vi "TDC_Prototype.vi"() -> ()   [LabVIEW 2025]
uses:
  Labview-File/STM-Auto-Project Testing/STM-Auto-Project (Trial 2)/QMH CTLS/Scan_Params (QMH).ctl
  TDC_SubVI/TEMP_SWEEPER.ctl
  TDC_SubVI/Temp Cntrl.ctl
  Downloads/OneDrive_2025-11-26 (2)/Magnetic Drift Correction/XY_Coords(Final).ctl
panel:
  out "Z-Controller on/off status 2":bool
  out "Translation (m) 2":T1
  out "Final coordinates (m)  2":cluster{"Xc":sgl, "Yc":sgl} {"Yc" format="%.4p"; "Xc" format="%.4p"}
  out "Initial coordinates (m)  2":cluster{"Xc":sgl, "Yc":sgl} {"Yc" format="%.4p"; "Xc" format="%.4p"}
  out "Current Temp":dbl format="%#.5f"
  out "Temp. Array":dbl[](array[numeric])
  out "Z-Controller on/off status":bool
  in  "Field and Temp Range":T2={"VISA (Magnet)"="COM4", "Fields(T)"=[], "Temps(K)"=[], "VISA (Temp) "="Lakeshore_Model_350"}
  out "error out":errorcluster
  in  "Serial Configuration":T3={"Baud Rate"=57600, "Parity"=1, "Data Bits"=7, "Stop Bits"=10, "Flow Control"=0}
  out "Current Index":i32
  out "Translation (m)":T1
  out "Final coordinates (m)":cluster{"Xc":sgl, "Yc":sgl} {"Yc" format="%.4p"; "Xc" format="%.4p"}
  out "Initial coordinates (m)":cluster{"Xc":sgl, "Yc":sgl} {"Yc" format="%.4p"; "Xc" format="%.4p"}
  in  "stop":bool
  in  "Start":bool
  # "Main goals,\n\nSet base line: Do initial bias and scan\n\nChange temp: Init temp, temp on, temp stab,\n\nInter scan, move frame, final scan, bias shit,\n\nNext temp? Prep next field though reinialization, determine if higher range is needed, apply field by changing setpoint\n\nInter scan, move frame, final scan, bias shit,"
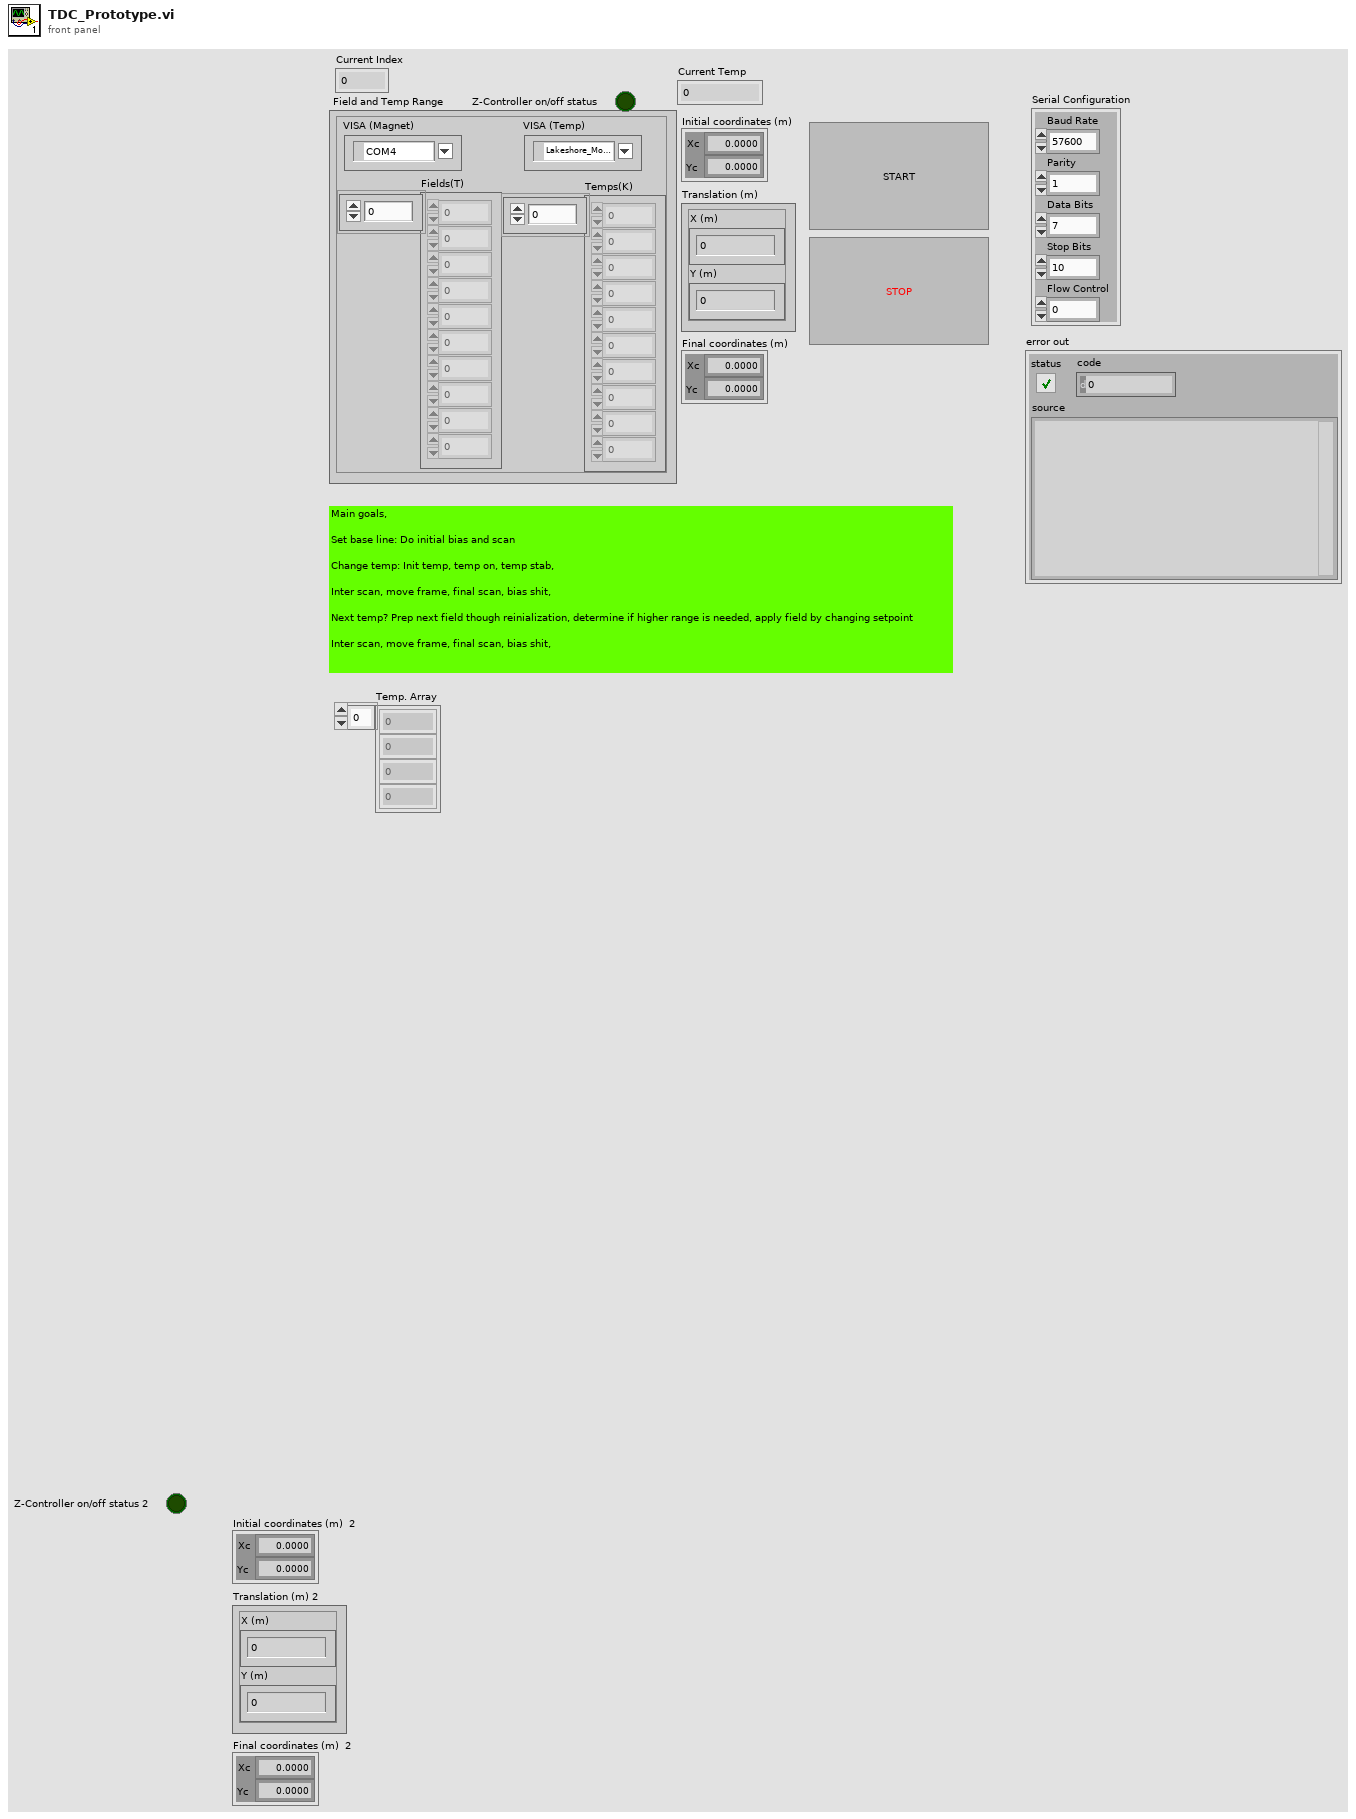
[diagram p1: front panel]
types:
  T1 = typedef "XY_Coords(Final).ctl" = cluster{"X (m)":dbl, "Y (m)":dbl}
  T2 = cluster{"VISA (Magnet)":refnum<visa-resource-name>, "Fields(T)":dbl[], "Temps(K)":dbl[], "VISA (Temp) ":refnum<visa-resource-name>}
  T3 = cluster{"Baud Rate":u32, "Parity":u16, "Data Bits":u16, "Stop Bits":u16, "Flow Control":u16}
  T4 = enum16{"1. BIAS", "2. INIT_SCAN", "3. SCAN_IDLE", "4. INTER_SCAN", "5. NEW_COORDS_&_FRAME", "6. FINAL_SCAN", "7. POLL_BIAS", "8. Z-CONT.", "9. STOP"}
  T5 = enum16{"SET TEMP", "SWEEP IDLE", "NEXT TEMP", "SWEEP DONE"}
  T6 = enum16{"1. INIT TEMP", "2. TC ON", "3. POLL_TEMPS", "4. TEMP_STAB", "5. TC IDLE", "6. APPLY NEXT TEMP", "7. TC OFF (Reset)"}
  T7 = typedef "Temp Cntrl.ctl" = cluster{"Range (0:Off)":u16, "Manual Output (0.00 %)":dbl, "Rate (D) (0.0 %)":dbl, "Reset (I) (20.0)":dbl, "Gain (P) (50.0)":dbl, "Power Up Enable (F: Disable)":bool, "Max User Current (2.000)":dbl, "Heater Resistance (1:25 Ohms)":u16, "Max Current (0:User Specified)":u16, "Heater Out Display (1:Current)":u16, "Mode (0:Off)":u16, "Input (0:None)":u16, "Target Temp (K)":dbl, "Serial Configuration":cluster{"Baud Rate":u32, "Parity":u16, "Data Bits":u16, "Stop Bits":u16, "Flow Control":u16}, "VISA resource name":refnum<visa-resource-name>, "Configure Control Parameters (0: Configure)":u16, "Enable Setpoint (F:Disable)":bool, "Input (0:A)":u16, "Data Source (0:Kelvin)":u16, "Output's Control Loop (1:1)":u16, "STND DEV Threshold ":dbl, "Mean Tolerance ":dbl, "Current State":enum16{"1. INIT TEMP", "2. TC ON", "3. POLL_TEMPS", "4. TEMP_STAB", "5. TC IDLE", "6. APPLY NEXT TEMP", "7. TC OFF (Reset)"}}
  T8 = typedef "TEMP_SWEEPER.ctl" = cluster{"Temps(K)":dbl[], "Sweep States":enum16{"SET TEMP", "SWEEP IDLE", "NEXT TEMP", "SWEEP DONE"}}
  T9 = typedef "Scan_Params (QMH).ctl" = cluster{"Setpoint (I)":dbl[], "Bias (V)":dbl[], "Number of scans":u8, "Port number (3364)":u32, "Avoid zero threshold (V)":dbl, "Current State":enum16{"1. BIAS", "2. INIT_SCAN", "3. SCAN_IDLE", "4. INTER_SCAN", "5. NEW_COORDS_&_FRAME", "6. FINAL_SCAN", "7. STOP"}}
  T10 = enum16{"1. BIAS", "2. INIT_SCAN", "3. SCAN_IDLE", "4. INTER_SCAN", "5. NEW_COORDS_&_FRAME", "6. FINAL_SCAN", "7. STOP"}
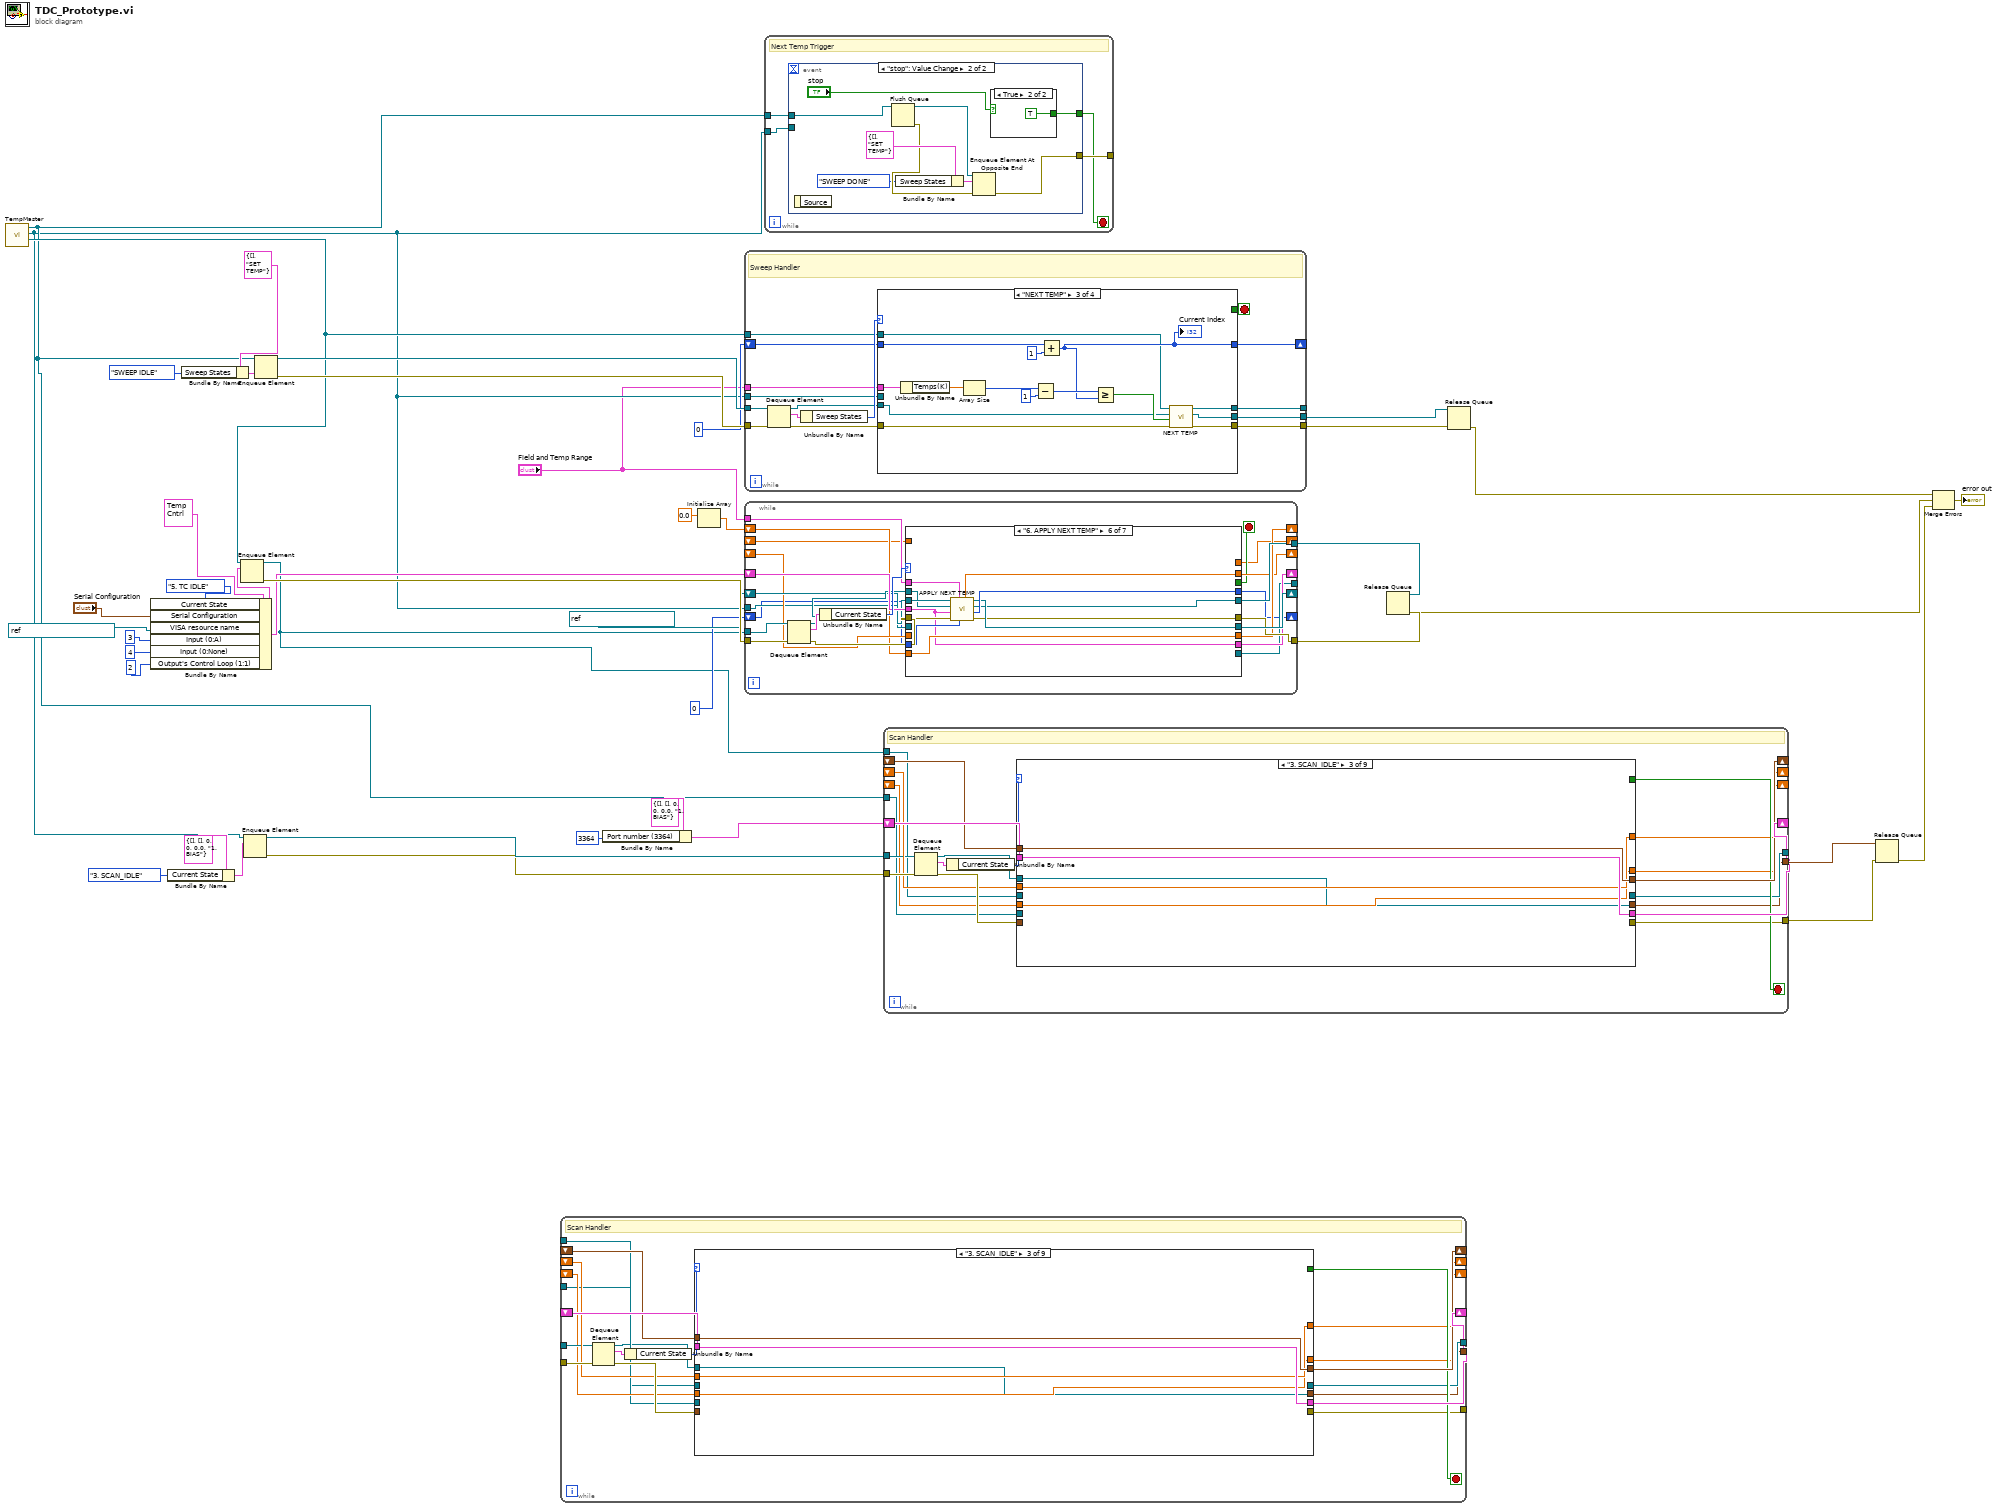
[diagram p0: block diagram]
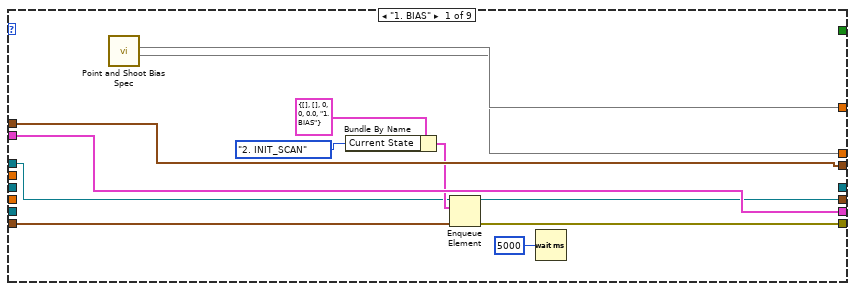
[diagram p2: hidden frame]
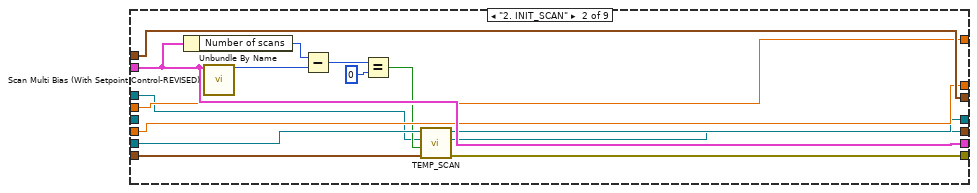
[diagram p3: hidden frame]
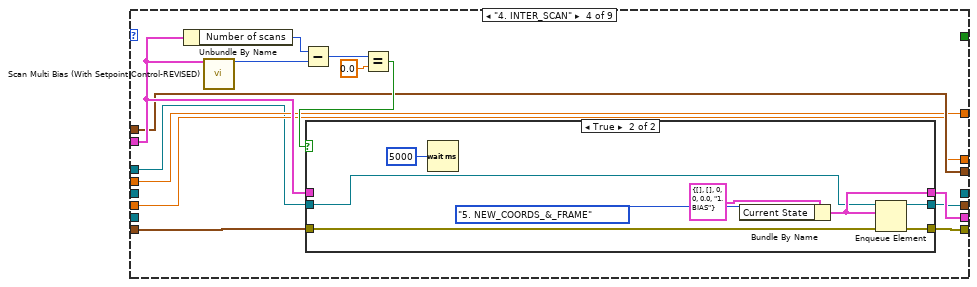
[diagram p4: hidden frame]
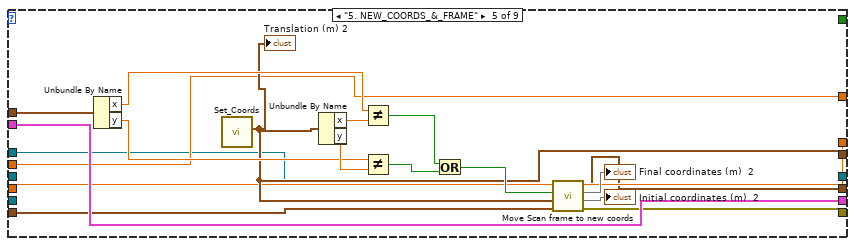
[diagram p6: hidden frame]
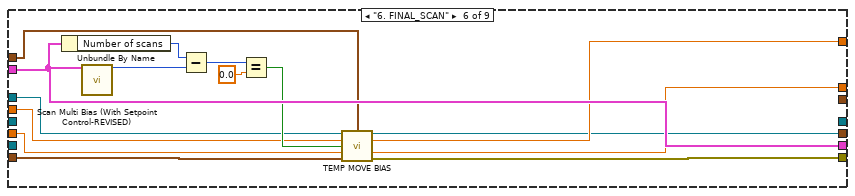
[diagram p7: hidden frame]
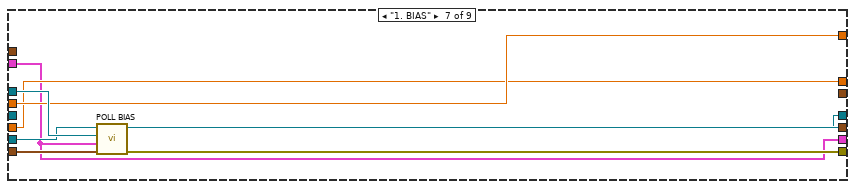
[diagram p8: hidden frame]
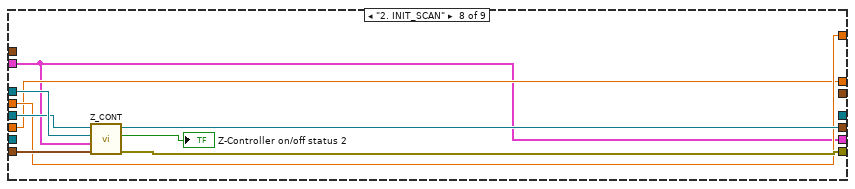
[diagram p9: hidden frame]
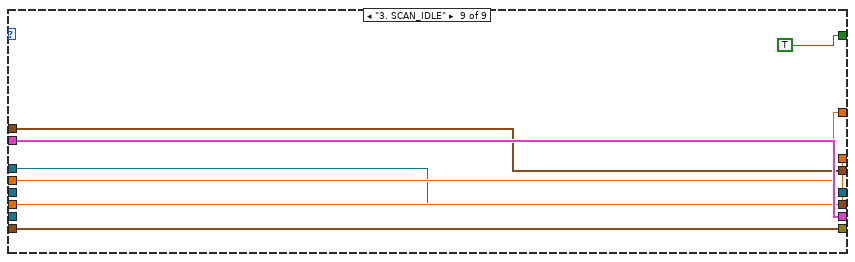
[diagram p10: hidden frame]
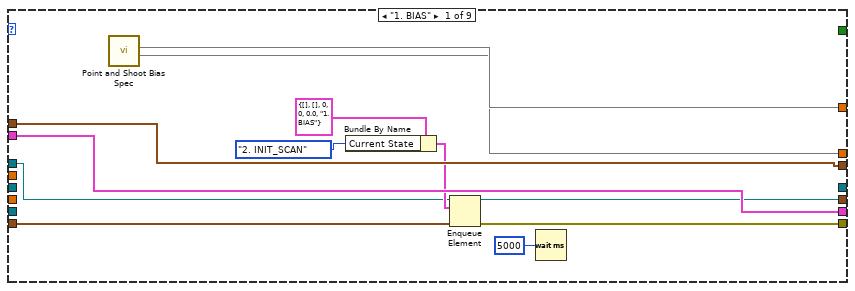
[diagram p11: hidden frame]
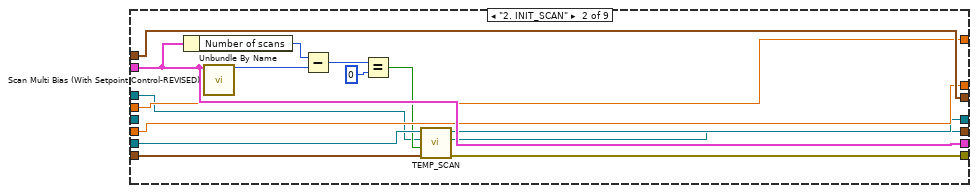
[diagram p12: hidden frame]
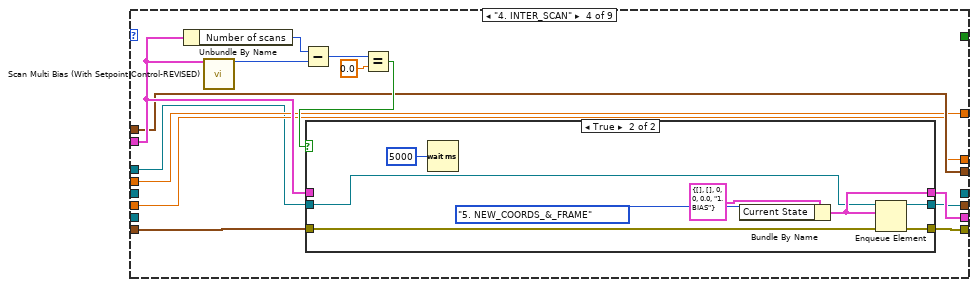
[diagram p13: hidden frame]
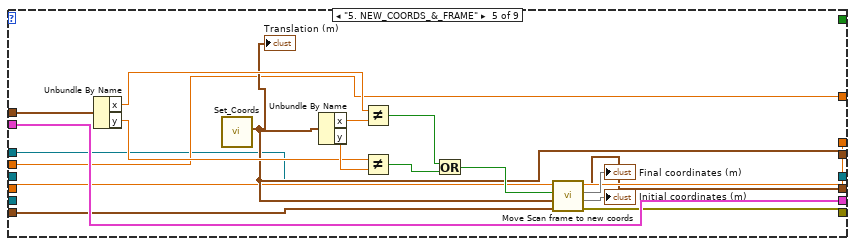
[diagram p15: hidden frame]
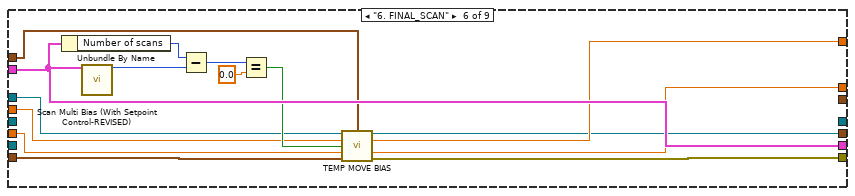
[diagram p16: hidden frame]
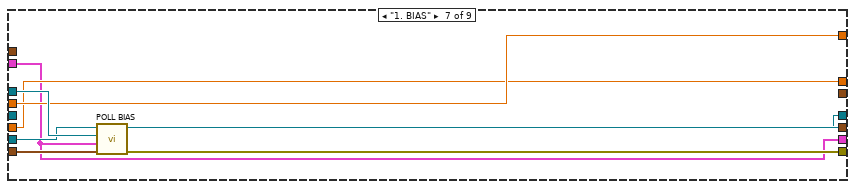
[diagram p17: hidden frame]
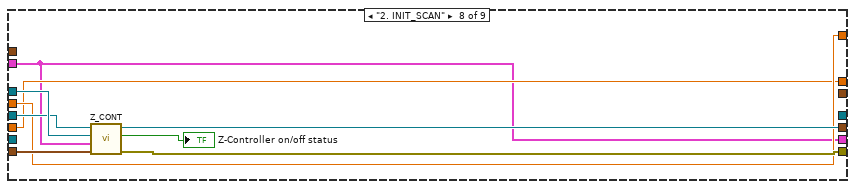
[diagram p18: hidden frame]
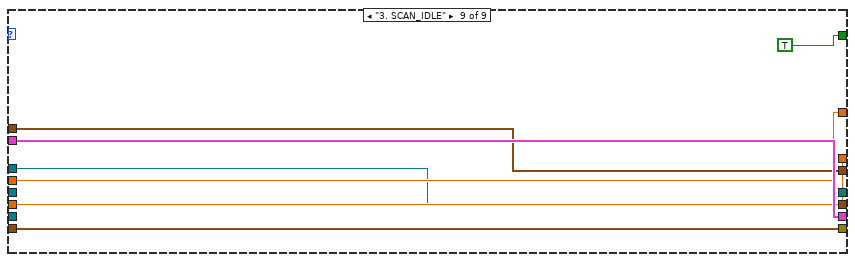
[diagram p19: hidden frame]
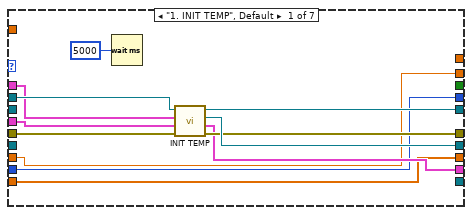
[diagram p20: hidden frame]
diagram:
  n1 = call "TempMaster.vi"() -> ("TempQ"=w27:refnum<queue>, "ScanQ"=w12:refnum<queue>, "SweepQ"=w17:refnum<queue>)  [unwired: 9 in]
  n2 = Bundle By Name(cluster=T7 {"Range (0:Off)"=0, "Manual Output (0.00 %)"=0.0, "Rate (D) (0.0 %)"=0.0, "Reset (I) (20.0)"=20.0, "Gain (P) (50.0)"=50.0, "Power Up Enable (F: Disable)"=FALSE, "Max User Current (2.000)"=2.0, "Heater Resistance (1:25 Ohms)"=1, "Max Current (0:User Specified)"=0, "Heater Out Display (1:Current)"=1, "Mode (0:Off)"=1, "Input (0:None)"=4, "Target Temp (K)"=5.0, "Serial Configuration"={"Baud Rate"=57600, "Parity"=1, "Data Bits"=7, "Stop Bits"=10, "Flow Control"=0}, "VISA resource name"="", "Configure Control Parameters (0: Configure)"=0, "Enable Setpoint (F:Disable)"=FALSE, "Input (0:A)"=3, "Data Source (0:Kelvin)"=0, "Output's Control Loop (1:1)"=2, "STND DEV Threshold "=0.1, "Mean Tolerance "=0.02, "Current State"=enum."1. INIT TEMP"} ("element"), "Current State"=T6."5. TC IDLE", "Serial Configuration"="Serial Configuration", "VISA resource name"=refnum<visa-resource-name> "Lakeshore_Model_350", "Input (0:A)"=u16 3, "Input (0:None)"=u16 4, "Output's Control Loop (1:1)"=u16 2) -> (w22:T7)
  n3 = Bundle By Name(cluster=T9 {"Setpoint (I)"=[], "Bias (V)"=[], "Number of scans"=0, "Port number (3364)"=0, "Avoid zero threshold (V)"=0.0, "Current State"=enum."1. BIAS"} ("element"), "Current State"=T4."3. SCAN_IDLE") -> (w37:T9)
  n4 = Bundle By Name(cluster=T8 {"Temps(K)"=[], "Sweep States"=enum."SET TEMP"} ("Temp and Field Range"), "Sweep States"=T5."SWEEP IDLE") -> (w41:T8)
  n5 = Enqueue Element(queue=w27, element=w22) -> (queue out=w2:refnum<queue>, error out=w28:errorcluster)  [unwired: 2 in, 1 out]
  n6 = Enqueue Element(queue=w12, element=w37) -> (queue out=w39:refnum<queue>, error out=w38:errorcluster)  [unwired: 2 in, 1 out]
  n7 = Enqueue Element(queue=w17, element=w41) -> (queue out=w42:refnum<queue>, error out=w40:errorcluster)  [unwired: 2 in, 1 out]
  n8 = while {
    tunnel: _ -> [w56]
    shift-right: [w61] -> _
    shift-left: _ -> [w62]
    shift-right: [w60] -> _
    shift-left: _ -> [w59]
    tunnel: [w57] -> _
    tunnel: [w54] -> _
    shift-right: [w52] -> _
    shift-left: _ -> [w53]
    tunnel: _ -> [w51]
    shift-right: [w48] -> _
    shift-left: _ -> [w47]
    tunnel: _ -> [w46]
    tunnel: [w45] -> _
    tunnel: _ -> [w43]
    stop <- w58 stop-if-true
    # "Scan Handler"
    n9 = Dequeue Element(queue=w51, error in (no error)=w56) -> (queue out=w44:refnum<queue>, element=w49:T9, error out=w55:errorcluster)  [unwired: 1 in, 1 out]
    n10 = Unbundle By Name(w49) -> ("Current State"=w50:T10)
    n11 = case shown="\"3. SCAN_IDLE\"" w50 {
      tunnel: w62 -> [w74 w86 w93 w102 w137 w149 w153 w162 w175]
      tunnel: w55 -> [w70 w79 _ w99 w127 w146 w161 w166 w176]
      tunnel: [w74 w86 w93 w103 w137 w149 w153 w162 w175] -> w61
      tunnel: [w73 w84 w94 w101 w124 _ _ _ w174] -> w60
      tunnel: w59 -> [w73 w84 w94 w101 w129 w144 _ _ w174]
      tunnel: [_ _ _ _ _ _ _ _ TRUE] -> w58
      tunnel: [w71 w75 _ w100 w128 w145 w156 w167 w176] -> w57
      tunnel: [_ w78 _ _ _ _ w157 _ _] -> w54
      tunnel: w53 -> [_ w83 w92 w98 w123 w142 w155 w164 w173]
      tunnel: [w64 w83 w92 w98 w123 w140 w155 w164 w173] -> w52
      tunnel: [w63 w82 w91 w97 w122 w139 w154 w163 w172] -> w48
      tunnel: w47 -> [_ w82 w91 w97 w122 w141 w154 w163 w172]
      tunnel: w46 -> [_ w81 _ _ _ _ w158 _ _]
      tunnel: [w66 w77 w90 w95 w120 w138 w159 w168 w171] -> w45
      tunnel: w44 -> [w67 w76 w90 w96 w121 w143 w160 w169 w171]
      tunnel: w43 -> [_ _ _ _ _ _ _ w165 _]
      frame "1. BIAS" {
        n12 = call "Point and Shoot Bias Spec.vi"() -> (1:w63, 2:w64)  [unwired: 9 in, 1 out]
        n13 = Bundle By Name(cluster=T9 {"Setpoint (I)"=[], "Bias (V)"=[], "Number of scans"=0, "Port number (3364)"=0, "Avoid zero threshold (V)"=0.0, "Current State"=enum."1. BIAS"} ("element"), "Current State"=T4."2. INIT_SCAN") -> (w68:T9)
        n14 = Enqueue Element(queue=w67, element=w68, error in (no error)=w70) -> (queue out=w66:refnum<queue>, error out=w71:errorcluster)  [unwired: 1 in, 1 out]
        n15 = Wait (ms)(milliseconds to wait=u32 5000) -> ()  [unwired: 1 out]
      }
      frame "2. INIT_SCAN" {
        n16 = Unbundle By Name(w86) -> ("Number of scans"=w85:u8)
        n17 = call "Scan Multi Bias (With Setpoint Control-REVISED).vi"("Scan Parameters"=w86) -> ("Scan"=w87:u8)  [unwired: 13 in, 1 out]
        n18 = Subtract(x=w85, y=w87) -> (x-y=w89:u8)
        n19 = Equal?(x=w89, y=u8 0) -> (x = y?=w80:bool)
        n20 = call "TEMP_SCAN.vi"("error in (no error)"=w79, "Boolean"=w80, "ScanQ in"=w76, "SweepQ in"=w81) -> ("error out"=w75:errorcluster, "ScanQ out"=w77:refnum<queue>, "SweepQ out"=w78:refnum<queue>)  [unwired: 5 in]
      }
      frame "3. SCAN_IDLE" {
      }
      frame "4. INTER_SCAN" {
        n21 = Unbundle By Name(w102) -> ("Number of scans"=w104:u8)
        n22 = call "Scan Multi Bias (With Setpoint Control-REVISED).vi"("Scan Parameters"=w102) -> ("Scan"=w105:u8)  [unwired: 13 in, 1 out]
        n23 = Subtract(x=w104, y=w105) -> (x-y=w107:u8)
        n24 = Equal?(x=w107, y=0.0) -> (x = y?=w106:bool)
        n25 = case shown="True" w106 {
          tunnel: [w111 w115] -> w103
          tunnel: w102 -> [w111 _]
          tunnel: [w110 w118] -> w100
          tunnel: w99 -> [w110 w117]
          tunnel: w96 -> [w109 w114]
          tunnel: [w109 w113] -> w95
          frame False {
          }
          frame True {
            n26 = Wait (ms)(milliseconds to wait=u32 5000) -> ()  [unwired: 1 out]
            n27 = Bundle By Name(cluster=T9 {"Setpoint (I)"=[], "Bias (V)"=[], "Number of scans"=0, "Port number (3364)"=0, "Avoid zero threshold (V)"=0.0, "Current State"=enum."1. BIAS"} ("element"), "Current State"=T4."5. NEW_COORDS_&_FRAME") -> (w115:T9)
            n28 = Enqueue Element(queue=w114, element=w115, error in (no error)=w117) -> (queue out=w113:refnum<queue>, error out=w118:errorcluster)  [unwired: 1 in, 1 out]
          }
        }
      }
      frame "5. NEW_COORDS_&_FRAME" {
        n29 = Unbundle By Name(w129) -> ("x"=w131:dbl, "y"=w130:dbl)
        n30 = call "Set_Coords.vi"() -> ("return value"=w124:cluster{"x":dbl, "y":dbl})  [unwired: 10 in, 1 out]
        "Translation (m) 2" <- w124
        n31 = Unbundle By Name(w124) -> ("x"=w134:dbl, "y"=w133:dbl)
        n32 = Not Equal?(x=w131, y=w134) -> (x != y?=w136:bool)
        n33 = Not Equal?(x=w130, y=w133) -> (x != y?=w135:bool)
        n34 = Or(x=w136, y=w135) -> (x .or. y?=w132:bool)
        n35 = call "Move Scan frame to new coords.vi"(9:w124, 10:w132, "Translation (m)"=w121) -> ("error out"=w128:errorcluster, 1:→"Initial coordinates (m)  2", 2:→"Final coordinates (m)  2", "Final coordinates (m)"=w120:cluster{"Xc":sgl, "Yc":sgl}, "Initial coordinates (m)"=w127:cluster{"Xc":sgl, "Yc":sgl})  [unwired: 4 in]
      }
      frame "6. FINAL_SCAN" {
        n36 = Unbundle By Name(w149) -> ("Number of scans"=w148:u8)
        n37 = call "Scan Multi Bias (With Setpoint Control-REVISED).vi"("Scan Parameters"=w149) -> ("Scan"=w150:u8)  [unwired: 13 in, 1 out]
        n38 = Subtract(x=w148, y=w150) -> (x-y=w151:u8)
        n39 = Equal?(x=w151, y=0.0) -> (x = y?=w147:bool)
        n40 = call "TEMP MOVE BIAS.vi"("ScanQ in"=w143, "Translation"=w144, "x"=w142, "Boolean"=w147, "y"=w141, "error in (no error)"=w146) -> ("ScanQ out"=w138:refnum<queue>, "X (m)"=w140:sgl, "Y (m)"=w139:sgl, "error out"=w145:errorcluster)  [unwired: 6 in]
      }
      frame "1. BIAS" {
        n41 = call "POLL BIAS.vi"("error in (no error)"=w161, "element"=w153, "ScanQ in"=w160, "Queue in"=w158) -> ("error out"=w156:errorcluster, "ScanQ out"=w159:refnum<queue>, "Queue out"=w157:refnum<queue>)  [unwired: 5 in]
      }
      frame "2. INIT_SCAN" {
        n42 = call "Z_CONT.vi"("error in (no error)"=w166, "element"=w162, "ScanQ in"=w169, "Queue in"=w165) -> ("error out"=w167:errorcluster, "Z-Controller on/off status"=→"Z-Controller on/off status 2":bool, "Queue out"=w168:refnum<queue>)  [unwired: 5 in]
      }
      frame "3. SCAN_IDLE" {
      }
    }
  }
  n43 = Bundle By Name(cluster=T9 {"Setpoint (I)"=[], "Bias (V)"=[], "Number of scans"=0, "Port number (3364)"=0, "Avoid zero threshold (V)"=0.0, "Current State"=enum."1. BIAS"} ("element"), "Port number (3364)"=u32 3364) -> (w34:T9)
  n44 = Initialize Array(0.0 ("element")) -> (w18:dbl[])  [unwired: 1 in]
  n45 = while {
    tunnel: w42 -> [w192]
    shift-right: [w185] -> _
    shift-left: 0 ("Current Index") -> [w186]
    tunnel: w27 -> [w184]
    tunnel: w40 -> [w191]
    tunnel: "Field and Temp Range" -> [w187]
    tunnel: [w183] -> w9
    tunnel: [w182] -> _
    tunnel: [w181] -> w8
    tunnel: w12 -> [w179]
    stop <- w178 stop-if-true
    # "Sweep Handler"
    n46 = Dequeue Element(queue=w192, error in (no error)=w191) -> (queue out=w188:refnum<queue>, element=w190:T8, error out=w180:errorcluster)  [unwired: 1 in, 1 out]
    n47 = Unbundle By Name(w190) -> ("Sweep States"=w189:T5)
    n48 = case shown="\"NEXT TEMP\"" w189 {
      tunnel: w188 -> [w206 w208 w215 w231]
      tunnel: w187 -> [_ _ w221 _]
      tunnel: w186 -> [w195 w210 w219 w229]
      tunnel: [w195 w210 w218 w229] -> w185
      tunnel: w184 -> [w198 w209 w216 w238]
      tunnel: [w201 w208 w211 w231] -> w183
      tunnel: [w197 w209 w212 w232] -> w182
      tunnel: [w196 w207 w214 w230] -> w181
      tunnel: w180 -> [w203 w207 w213 _]
      tunnel: w179 -> [_ _ _ w236]
      tunnel: [_ _ _ TRUE] -> w178
      frame "SET TEMP" {
        n49 = Bundle By Name(cluster=T8 {"Temps(K)"=[], "Sweep States"=enum."SET TEMP"} ("Temp and Field Range"), "Sweep States"=T5."SWEEP IDLE") -> (w204:T8)
        n50 = Bundle By Name(cluster=T7 {"Range (0:Off)"=0, "Manual Output (0.00 %)"=0.0, "Rate (D) (0.0 %)"=0.0, "Reset (I) (20.0)"=20.0, "Gain (P) (50.0)"=50.0, "Power Up Enable (F: Disable)"=FALSE, "Max User Current (2.000)"=2.0, "Heater Resistance (1:25 Ohms)"=1, "Max Current (0:User Specified)"=0, "Heater Out Display (1:Current)"=1, "Mode (0:Off)"=1, "Input (0:None)"=4, "Target Temp (K)"=5.0, "Serial Configuration"={"Baud Rate"=57600, "Parity"=1, "Data Bits"=7, "Stop Bits"=10, "Flow Control"=0}, "VISA resource name"="", "Configure Control Parameters (0: Configure)"=0, "Enable Setpoint (F:Disable)"=FALSE, "Input (0:A)"=3, "Data Source (0:Kelvin)"=0, "Output's Control Loop (1:1)"=2, "STND DEV Threshold "=0.1, "Mean Tolerance "=0.02, "Current State"=enum."1. INIT TEMP"} ("element"), "Current State"=T6."1. INIT TEMP") -> (w199:T7)
        n51 = Enqueue Element(queue=w206, element=w204, error in (no error)=w203) -> (queue out=w201:refnum<queue>, error out=w202:errorcluster)  [unwired: 1 in, 1 out]
        n52 = Enqueue Element(queue=w198, element=w199, error in (no error)=w202) -> (queue out=w197:refnum<queue>, error out=w196:errorcluster)  [unwired: 1 in, 1 out]
      }
      frame "SWEEP IDLE" {
      }
      frame "NEXT TEMP" {
        n53 = Unbundle By Name(w221) -> ("Temps(K)"=w220:dbl[])
        n54 = Array Size(array=w220) -> (size(s)=w224:i32)
        n55 = Subtract(x=w224, y=1) -> (x-y=w222:i32)
        n56 = Add(x=w219, y=1) -> (x+y=w218:i32)
        "Current Index" <- w218
        n57 = Greater Or Equal?(x=w222, y=w218) -> (x >= y?=w217:bool)
        n58 = call "NEXT TEMP.vi"("error in (no error)"=w213, "Boolean"=w217, "SweepQ"=w215, "TempQ"=w216) -> ("error out"=w214:errorcluster, "SweepQ Out"=w211:refnum<queue>, "TEMPQ Out"=w212:refnum<queue>)  [unwired: 5 in]
      }
      frame "SWEEP DONE" {
        n59 = Bundle By Name(cluster=T9 {"Setpoint (I)"=[], "Bias (V)"=[], "Number of scans"=0, "Port number (3364)"=0, "Avoid zero threshold (V)"=0.0, "Current State"=enum."1. BIAS"} ("element"), "Current State"=T4."9. STOP") -> (w235:T9)
        n60 = Bundle By Name(cluster=T7 {"Range (0:Off)"=0, "Manual Output (0.00 %)"=0.0, "Rate (D) (0.0 %)"=0.0, "Reset (I) (20.0)"=20.0, "Gain (P) (50.0)"=50.0, "Power Up Enable (F: Disable)"=FALSE, "Max User Current (2.000)"=2.0, "Heater Resistance (1:25 Ohms)"=1, "Max Current (0:User Specified)"=0, "Heater Out Display (1:Current)"=1, "Mode (0:Off)"=1, "Input (0:None)"=4, "Target Temp (K)"=5.0, "Serial Configuration"={"Baud Rate"=57600, "Parity"=1, "Data Bits"=7, "Stop Bits"=10, "Flow Control"=0}, "VISA resource name"="", "Configure Control Parameters (0: Configure)"=0, "Enable Setpoint (F:Disable)"=FALSE, "Input (0:A)"=3, "Data Source (0:Kelvin)"=0, "Output's Control Loop (1:1)"=2, "STND DEV Threshold "=0.1, "Mean Tolerance "=0.02, "Current State"=enum."1. INIT TEMP"} ("element"), "Current State"=T6."7. TC OFF (Reset)") -> (w233:T7)
        n61 = Enqueue Element(queue=w236, element=w235) -> (error out=w239:errorcluster)  [unwired: 2 in, 2 out]
        n62 = Enqueue Element At Opposite End(queue=w238, element=w233, error in (no error)=w239) -> (queue out=w232:refnum<queue>, error out=w230:errorcluster)  [unwired: 1 in, 1 out]
      }
    }
  }
  n63 = while {
    tunnel: w2 -> [w263]
    tunnel: w28 -> [w262]
    shift-right: [w252] -> _
    shift-left: w22 -> [w259]
    tunnel: "Field and Temp Range" -> [w257]
    shift-right: [w256] -> _
    shift-left: refnum<visa-resource-name> "Lakeshore_Model_350" ("VISA resource name out") -> [w251]
    tunnel: [w255] -> w10
    tunnel: [w253] -> w11
    shift-right: [w247] -> _
    shift-left: _ -> [w250]
    shift-right: [w248] -> _
    shift-left: w18 -> [w249]
    tunnel: w12 -> [w246]
    tunnel: [w245] -> _
    shift-right: [w243] -> _
    shift-left: 0 -> [w244]
    shift-right: [w241] -> _
    shift-left: _ -> [w240]
    stop <- w242 stop-if-true
    n64 = Dequeue Element(queue=w263, error in (no error)=w262) -> (queue out=w254:refnum<queue>, element=w261:T7, error out=w258:errorcluster)  [unwired: 1 in, 1 out]
    n65 = Unbundle By Name(w261) -> ("Current State"=w260:T6)
    n66 = case shown="\"6. APPLY NEXT TEMP\"" w260 {
      tunnel: w259 -> [w275 w289 w297 w314 w318 w325 w342]
      tunnel: w258 -> [w274 w283 w301 w313 w319 w331 w345]
      tunnel: w257 -> [w264 w282 _ _ _ w326 _]
      tunnel: [w273 w281 w300 w304 w320 w330 w344] -> w256
      tunnel: [w270 w286 w292 w311 w319 w327 w341] -> w255
      tunnel: w254 -> [w272 w288 w294 w315 w321 w329 w343]
      tunnel: [w271 w287 w293 w312 w321 w328 w340] -> w253
      tunnel: [w268 w285 w297 w308 w318 w325 w339] -> w252
      tunnel: w251 -> [_ w284 w302 w304 w320 w332 w346]
      tunnel: [w266 w280 w299 w309 w322 w324 w337] -> w247
      tunnel: w250 -> [w266 _ w299 w309 w322 _ w337]
      tunnel: w249 -> [w267 w279 w290 w316 w323 w335 w347]
      tunnel: [w267 w279 w290 w310 w323 w335 w347] -> w248
      tunnel: w246 -> [_ w277 _ w307 _ _ _]
      tunnel: [_ w276 _ w306 _ _ _] -> w245
      tunnel: w244 -> [w265 w278 w298 w305 w317 w334 w338]
      tunnel: [w265 w278 w298 w305 w317 w333 w338] -> w243
      tunnel: [_ _ _ _ _ _ TRUE] -> w242
      tunnel: [_ _ w291 _ _ _ _] -> w241
      tunnel: w240 -> [_ _ _ w303 _ _ _]
      frame "1. INIT TEMP", Default {
        n67 = Wait (ms)(milliseconds to wait=u32 5000) -> ()  [unwired: 1 out]
        n68 = call "INIT TEMP.vi"("error in (no error)"=w274, "element"=w275, "Field and Temp Range"=w264, "Queue in"=w272) -> ("error out"=w270:errorcluster, "output cluster"=w268:T7, "VISA resource name out"=w273:refnum<visa-resource-name>, "Queue out"=w271:refnum<queue>)  [unwired: 4 in]
      }
      frame "2. TC ON" {
        n69 = call "TEMP ON.vi"("ScanQ in"=w277, "element in"=w289, "error in (no error)"=w283, "Field and Temp Range"=w282, "TempQ in"=w288, "VISA Refnum in"=w284) -> ("error out"=w286:errorcluster, "element out"=w285:T7, "TempQ out"=w287:refnum<queue>, "VISA Refnum out"=w281:refnum<visa-resource-name>, "ScanQ out"=w276:refnum<queue>, "Setpoint"=w280:dbl)
      }
      frame "3. POLL_TEMPS" {
        n70 = call "POLL TEMP.vi"("element"=w297, "error in (no error)"=w301, "VISA resource name in"=w302) -> ("VISA resource name out"=w300:refnum<visa-resource-name>, "Sensor Data"=w291:dbl)  [unwired: 7 in]
        "Current Temp" <- w291
        n71 = Bundle By Name(cluster=w297, "Current State"=T6."4. TEMP_STAB") -> (w296:T7)
        n72 = Enqueue Element(queue=w294, element=w296) -> (queue out=w293:refnum<queue>, error out=w292:errorcluster)  [unwired: 2 in, 1 out]
      }
      frame "4. TEMP_STAB" {
        n73 = call "TEMP STAB.vi"("Queue in"=w315, "element in"=w314, "element 2"=w316, "ScanQ In"=w307, "Setpoint"=w309, "error in (no error)"=w313, "element"=w303) -> ("Queue out"=w312:refnum<queue>, "Array out"=w310:dbl[], "ScanQ"=w306:refnum<queue>, "element out"=w308:T7, "error out"=w311:errorcluster)  [unwired: 4 in]
        "Temp. Array" <- w310
      }
      frame "5. TC IDLE" {
      }
      frame "6. APPLY NEXT TEMP" {
        n74 = call "APPLY NEXT TEMP.vi"("Numeric in"=w334, "Field and Temp Range"=w326, "error in (no error)"=w331, "element in"=w325, "TempQ in"=w329, "VISA Refnum in"=w332) -> ("error out"=w327:errorcluster, "Numeric out"=w333:i32, "TempQ out"=w328:refnum<queue>, "VISA Refnum out"=w330:refnum<visa-resource-name>, "New SP"=w324:dbl)  [unwired: 1 in]
      }
      frame "7. TC OFF (Reset)" {
        n75 = call "TEMP OFF.vi"("error in (no error)"=w345, "element in"=w342, "TempQ in"=w343, "VISA Refnum in"=w346) -> ("error out"=w341:errorcluster, "element out"=w339:T7, "TempQ out"=w340:refnum<queue>, "VISA Refnum out"=w344:refnum<visa-resource-name>)  [unwired: 4 in]
      }
    }
  }
  n76 = while {
    tunnel: [w351] -> _
    tunnel: w17 -> [w349]
    tunnel: w12 -> [w348]
    stop <- w350 stop-if-true
    # "Next Temp Trigger"
    n77 = event shown="[1] \"stop\": Value Change" {
      selector: _ -> [_ _]
      dyn-events: _ -> [_ _]
      timeout: _ -> [_ _]
      tunnel: [w356 w365] -> w351
      tunnel: [_ w363] -> w350
      tunnel: w349 -> [_ w360]
      tunnel: w348 -> [w354 _]
      event "Start": Value Change {
        n78 = event-data() -> ()  [unwired: 1 in, 1 out]
        n79 = Bundle By Name(cluster=T9 {"Setpoint (I)"=[], "Bias (V)"=[], "Number of scans"=0, "Port number (3364)"=0, "Avoid zero threshold (V)"=0.0, "Current State"=enum."1. BIAS"} ("element"), "Current State"=T4."1. BIAS") -> (w353:T9)
        n80 = Enqueue Element(queue=w354, element=w353) -> (error out=w356:errorcluster)  [unwired: 2 in, 2 out]
      }
      event "stop": Value Change {
        n81 = event-data() -> ()  [unwired: 1 in, 1 out]
        n82 = Flush Queue(queue=w360) -> (queue out=w359:refnum<queue>, error out=w358:errorcluster)  [unwired: 1 in, 1 out]
        n83 = Bundle By Name(cluster=T8 {"Temps(K)"=[], "Sweep States"=enum."SET TEMP"} ("Temp and Field Range"), "Sweep States"=T5."SWEEP DONE") -> (w361:T8)
        n84 = Enqueue Element At Opposite End(queue=w359, element=w361, error in (no error)=w358) -> (error out=w365:errorcluster)  [unwired: 1 in, 2 out]
        n85 = case shown="True" "stop" {
          tunnel: [FALSE ("stop 2") TRUE ("stop 2")] -> w363
          frame False {
          }
          frame True {
          }
        }
      }
    }
  }
  n86 = while {
    tunnel: w38 -> [w381]
    shift-right: [w386] -> _
    shift-left: w34 -> [w387]
    shift-right: [w385] -> _
    shift-left: _ -> [w384]
    tunnel: [w382] -> w36
    tunnel: [w379] -> _
    shift-right: [w377] -> _
    shift-left: _ -> [w378]
    tunnel: w39 -> [w376]
    shift-right: [w373] -> _
    shift-left: _ -> [w372]
    tunnel: w17 -> [w371]
    tunnel: [w370] -> w16
    tunnel: w2 -> [w368]
    stop <- w383 stop-if-true
    # "Scan Handler"
    n87 = Dequeue Element(queue=w376, error in (no error)=w381) -> (queue out=w369:refnum<queue>, element=w374:T9, error out=w380:errorcluster)  [unwired: 1 in, 1 out]
    n88 = Unbundle By Name(w374) -> ("Current State"=w375:T10)
    n89 = case shown="\"3. SCAN_IDLE\"" w375 {
      tunnel: w387 -> [w399 w411 w418 w427 w462 w474 w478 w487 w500]
      tunnel: w380 -> [w395 w404 _ w424 w452 w471 w486 w491 w501]
      tunnel: [w399 w411 w418 w428 w462 w474 w478 w487 w500] -> w386
      tunnel: [w398 w409 w419 w426 w449 _ _ _ w499] -> w385
      tunnel: w384 -> [w398 w409 w419 w426 w454 w469 _ _ w499]
      tunnel: [_ _ _ _ _ _ _ _ TRUE] -> w383
      tunnel: [w396 w400 _ w425 w453 w470 w481 w492 w501] -> w382
      tunnel: [_ w403 _ _ _ _ w482 _ _] -> w379
      tunnel: w378 -> [_ w408 w417 w423 w448 w467 w480 w489 w498]
      tunnel: [w389 w408 w417 w423 w448 w465 w480 w489 w498] -> w377
      tunnel: [w388 w407 w416 w422 w447 w464 w479 w488 w497] -> w373
      tunnel: w372 -> [_ w407 w416 w422 w447 w466 w479 w488 w497]
      tunnel: w371 -> [_ w406 _ _ _ _ w483 _ _]
      tunnel: [w391 w402 w415 w420 w445 w463 w484 w493 w496] -> w370
      tunnel: w369 -> [w392 w401 w415 w421 w446 w468 w485 w494 w496]
      tunnel: w368 -> [_ _ _ _ _ _ _ w490 _]
      frame "1. BIAS" {
        n90 = call "Point and Shoot Bias Spec.vi"() -> (1:w388, 2:w389)  [unwired: 9 in, 1 out]
        n91 = Bundle By Name(cluster=T9 {"Setpoint (I)"=[], "Bias (V)"=[], "Number of scans"=0, "Port number (3364)"=0, "Avoid zero threshold (V)"=0.0, "Current State"=enum."1. BIAS"} ("element"), "Current State"=T4."2. INIT_SCAN") -> (w393:T9)
        n92 = Enqueue Element(queue=w392, element=w393, error in (no error)=w395) -> (queue out=w391:refnum<queue>, error out=w396:errorcluster)  [unwired: 1 in, 1 out]
        n93 = Wait (ms)(milliseconds to wait=u32 5000) -> ()  [unwired: 1 out]
      }
      frame "2. INIT_SCAN" {
        n94 = Unbundle By Name(w411) -> ("Number of scans"=w410:u8)
        n95 = call "Scan Multi Bias (With Setpoint Control-REVISED).vi"("Scan Parameters"=w411) -> ("Scan"=w412:u8)  [unwired: 13 in, 1 out]
        n96 = Subtract(x=w410, y=w412) -> (x-y=w414:u8)
        n97 = Equal?(x=w414, y=u8 0) -> (x = y?=w405:bool)
        n98 = call "TEMP_SCAN.vi"("error in (no error)"=w404, "Boolean"=w405, "ScanQ in"=w401, "SweepQ in"=w406) -> ("error out"=w400:errorcluster, "ScanQ out"=w402:refnum<queue>, "SweepQ out"=w403:refnum<queue>)  [unwired: 5 in]
      }
      frame "3. SCAN_IDLE" {
      }
      frame "4. INTER_SCAN" {
        n99 = Unbundle By Name(w427) -> ("Number of scans"=w429:u8)
        n100 = call "Scan Multi Bias (With Setpoint Control-REVISED).vi"("Scan Parameters"=w427) -> ("Scan"=w430:u8)  [unwired: 13 in, 1 out]
        n101 = Subtract(x=w429, y=w430) -> (x-y=w432:u8)
        n102 = Equal?(x=w432, y=0.0) -> (x = y?=w431:bool)
        n103 = case shown="True" w431 {
          tunnel: [w436 w440] -> w428
          tunnel: w427 -> [w436 _]
          tunnel: [w435 w443] -> w425
          tunnel: w424 -> [w435 w442]
          tunnel: w421 -> [w434 w439]
          tunnel: [w434 w438] -> w420
          frame False {
          }
          frame True {
            n104 = Wait (ms)(milliseconds to wait=u32 5000) -> ()  [unwired: 1 out]
            n105 = Bundle By Name(cluster=T9 {"Setpoint (I)"=[], "Bias (V)"=[], "Number of scans"=0, "Port number (3364)"=0, "Avoid zero threshold (V)"=0.0, "Current State"=enum."1. BIAS"} ("element"), "Current State"=T4."5. NEW_COORDS_&_FRAME") -> (w440:T9)
            n106 = Enqueue Element(queue=w439, element=w440, error in (no error)=w442) -> (queue out=w438:refnum<queue>, error out=w443:errorcluster)  [unwired: 1 in, 1 out]
          }
        }
      }
      frame "5. NEW_COORDS_&_FRAME" {
        n107 = Unbundle By Name(w454) -> ("x"=w456:dbl, "y"=w455:dbl)
        n108 = call "Set_Coords.vi"() -> ("return value"=w449:cluster{"x":dbl, "y":dbl})  [unwired: 10 in, 1 out]
        "Translation (m)" <- w449
        n109 = Unbundle By Name(w449) -> ("x"=w459:dbl, "y"=w458:dbl)
        n110 = Not Equal?(x=w456, y=w459) -> (x != y?=w461:bool)
        n111 = Not Equal?(x=w455, y=w458) -> (x != y?=w460:bool)
        n112 = Or(x=w461, y=w460) -> (x .or. y?=w457:bool)
        n113 = call "Move Scan frame to new coords.vi"(9:w449, 10:w457, "Translation (m)"=w446) -> ("error out"=w453:errorcluster, 1:→"Initial coordinates (m)", 2:→"Final coordinates (m)", "Final coordinates (m)"=w445:cluster{"Xc":sgl, "Yc":sgl}, "Initial coordinates (m)"=w452:cluster{"Xc":sgl, "Yc":sgl})  [unwired: 4 in]
      }
      frame "6. FINAL_SCAN" {
        n114 = Unbundle By Name(w474) -> ("Number of scans"=w473:u8)
        n115 = call "Scan Multi Bias (With Setpoint Control-REVISED).vi"("Scan Parameters"=w474) -> ("Scan"=w475:u8)  [unwired: 13 in, 1 out]
        n116 = Subtract(x=w473, y=w475) -> (x-y=w476:u8)
        n117 = Equal?(x=w476, y=0.0) -> (x = y?=w472:bool)
        n118 = call "TEMP MOVE BIAS.vi"("ScanQ in"=w468, "Translation"=w469, "x"=w467, "Boolean"=w472, "y"=w466, "error in (no error)"=w471) -> ("ScanQ out"=w463:refnum<queue>, "X (m)"=w465:sgl, "Y (m)"=w464:sgl, "error out"=w470:errorcluster)  [unwired: 6 in]
      }
      frame "1. BIAS" {
        n119 = call "POLL BIAS.vi"("error in (no error)"=w486, "element"=w478, "ScanQ in"=w485, "Queue in"=w483) -> ("error out"=w481:errorcluster, "ScanQ out"=w484:refnum<queue>, "Queue out"=w482:refnum<queue>)  [unwired: 5 in]
      }
      frame "2. INIT_SCAN" {
        n120 = call "Z_CONT.vi"("error in (no error)"=w491, "element"=w487, "ScanQ in"=w494, "Queue in"=w490) -> ("error out"=w492:errorcluster, "Z-Controller on/off status"=→"Z-Controller on/off status":bool, "Queue out"=w493:refnum<queue>)  [unwired: 5 in]
      }
      frame "3. SCAN_IDLE" {
      }
    }
  }
  n121 = Release Queue(queue=w11, error in (no error)=w10) -> (error out=w6:errorcluster)  [unwired: 1 in, 2 out]
  n122 = Release Queue(queue=w9, error in (no error)=w8) -> (error out=w7:errorcluster)  [unwired: 1 in, 2 out]
  n123 = Release Queue(queue=w16, error in (no error)=w36) -> (error out=w5:errorcluster)  [unwired: 1 in, 2 out]
  n124 = Merge Errors(w7, w6, w5) -> (→"error out":errorcluster)
